vi "GenerateTriggeredStimulus.vi"(8 "error in (no error)":errorcluster, 11 "Stimulus in":refnum<class "TriggerOnTurnsTwoColors.lvclass">) -> (0 "error out":errorcluster, 2 "TriggeredStimulus":sgl[][](array[numeric]), 3 "Stimulus out":refnum<class "TriggerOnTurnsTwoColors.lvclass">)   [LabVIEW 2019, in "TriggerOnTurnsTwoColors.lvclass"]
uses:
  TriggerOnTurnsTwoColors.lvclass
  TriggerOnTurnsTwoColors.lvclass/TriggerOnTurnsTwoColors.ctl
  <vilib>/numeric/Random Number (Range) U64.vi
  <vilib>/numeric/sub_Random U32.vi
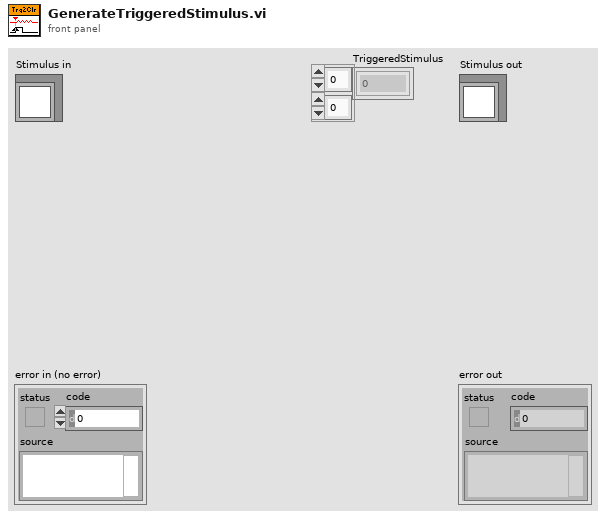
[diagram p1: front panel]
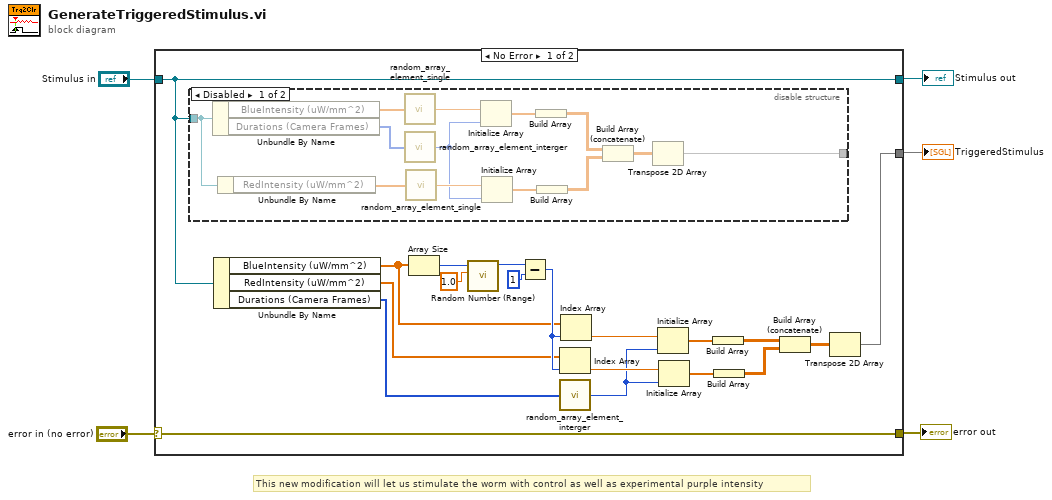
[diagram p0: block diagram]
diagram:
  # "This new modification will let us stimulate the worm with control as well as experimental purple intensity"
  n1 = case shown="No Error" "error in (no error)" {
    selector: "error in (no error)" -> [w24 w39]
    tunnel: [w24 w39] -> w1
    tunnel: [w19 w38] -> w3
    tunnel: "Stimulus in" -> [w19 w38]
    tunnel: [w6 _] -> w2
    frame No Error {
      n2 = disable-structure shown="Disabled" {
        disable-tunnel: w19 -> [w26 _]
        disable-tunnel: [w25 _] -> _
        frame Disabled {
          n3 = Unbundle By Name(w26) -> ("BlueIntensity (uW/mm^2)"=w37:sgl[], "Durations (Camera Frames)"=w28:i32[])
          n4 = Unbundle By Name(w26) -> ("RedIntensity (uW/mm^2)"=w33:sgl[])
          n5 = call "random_array_element_single.vi"("Array of numbers"=w37) -> ("Randomly selected number"=w36:sgl)
          n6 = call "random_array_element_interger.vi"("Array of numbers"=w28) -> ("Randomly selected number"=w27:i32)
          n7 = call "random_array_element_single.vi"("Array of numbers"=w33) -> ("Randomly selected number"=w32:sgl)
          n8 = Initialize Array(w36, w27) -> (w35:sgl[])
          n9 = Initialize Array(w32, w27) -> (w34:sgl[])
          n10 = Build Array(w35) -> (w30:sgl[][])
          n11 = Build Array(w34) -> (w29:sgl[][])
          n12 = Build Array (concatenate)(w30, w29) -> (w31:sgl[][])
          n13 = Transpose 2D Array(2D array=w31) -> (transposed array=w25:sgl[][])
        }
        frame Enabled {
        }
      }
      n14 = Unbundle By Name(w19) -> ("BlueIntensity (uW/mm^2)"=w9:sgl[], "RedIntensity (uW/mm^2)"=w8:sgl[], "Durations (Camera Frames)"=w7:i32[])
      n15 = Array Size(array=w9) -> (size(s)=w23:i32)
      n16 = call-poly <vilib>:"Random Number (Range).vi"("lower bound (0)"=1.0, "upper bound (100)"=w23) -> ("number"=w21:u64)  [unwired: 9 in]
      n17 = Subtract(x=w21, y=u64 1) -> (x-y=w10:u64)
      n18 = Index Array(array=w8, index=w10) -> (element=w12:sgl)
      n19 = call "random_array_element_interger.vi"("Array of numbers"=w7) -> ("Randomly selected number"=w11:i32)
      n20 = Index Array(array=w9, index=w10) -> (element=w13:sgl)
      n21 = Initialize Array(w13, w11) -> (w18:sgl[])
      n22 = Initialize Array(w12, w11) -> (w17:sgl[])
      n23 = Build Array(w18) -> (w15:sgl[][])
      n24 = Build Array(w17) -> (w14:sgl[][])
      n25 = Build Array (concatenate)(w15, w14) -> (w16:sgl[][])
      n26 = Transpose 2D Array(2D array=w16) -> (transposed array=w6:sgl[][])
    }
    frame Error {
    }
  }
  "error out" <- w1
  "Stimulus out" <- w3
  "TriggeredStimulus" <- w2
